vi "NK11003_Config.vi"(7 "频率":enum16{"50HZ", "60HZ"}(ring), 8 "error in":errorcluster caption="错误输入（无错误）", 9 "电流":dbl=10.0 min=1.0 max=13.0 format="%#_4f", 10 "电压":dbl=220.0 min=1.0 max=300.0 format="%#_4f", 11 "MyIndex":u8) -> (0 "error out":errorcluster, 3 "OK?":bool)   [LabVIEW 2015]
uses:
  <vilib>/Instr/_visa.llb/VISA Configure Serial Port (Instr).vi
panel:
  out "VISA":refnum<visa-resource-name> caption="VISA资源名称输出"
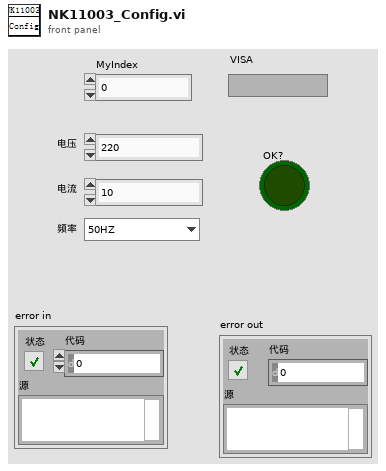
[diagram p1: front panel]
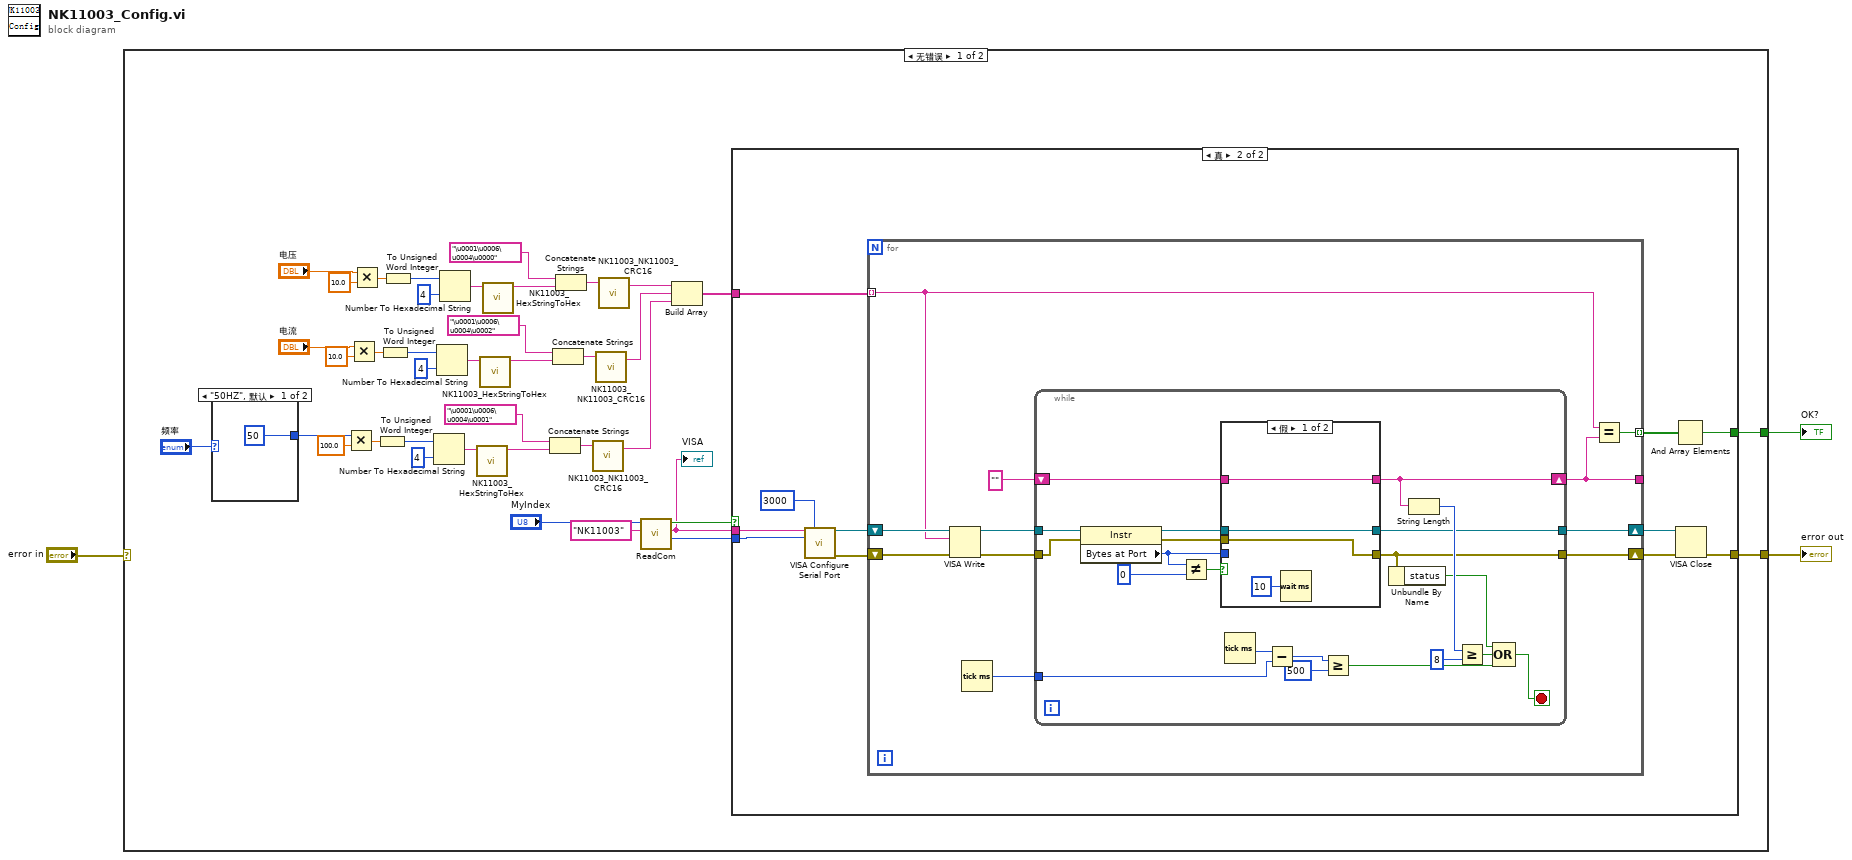
[diagram p0: block diagram]
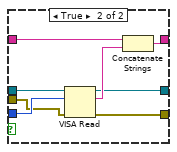
[diagram p3: hidden frame]
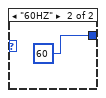
[diagram p4: hidden frame]
diagram:
  n1 = case shown="无错误" "error in" {
    selector: "error in" -> [_ w100]
    tunnel: [w8 _] -> w3
    tunnel: [w4 w100] -> w2
    frame No Error {
      n2 = case shown="\"50HZ\", 默认" "频率" {
        tunnel: [50 60] -> w14
        frame "50HZ", Default {
        }
        frame "60HZ" {
        }
      }
      n3 = Multiply(x=w14, y=100.0) -> (x*y=w21:dbl)
      n4 = Multiply(x="电流", y=10.0) -> (x*y=w27:dbl)
      n5 = Multiply(x="电压", y=10.0) -> (x*y=w38:dbl)
      n6 = To Unsigned Word Integer(number=w21) -> (unsigned 16bit integer=w20:u16)
      n7 = To Unsigned Word Integer(number=w27) -> (unsigned 16bit integer=w28:u16)
      n8 = To Unsigned Word Integer(number=w38) -> (unsigned 16bit integer=w37:u16)
      n9 = Number To Hexadecimal String(1:i16 4 ("宽度(-)"), 2:w20) -> (0:w18:string)
      n10 = Number To Hexadecimal String(1:i16 4 ("宽度(-)"), 2:w28) -> (0:w30:string)
      n11 = Number To Hexadecimal String(1:i16 4 ("宽度(-)"), 2:w37) -> (0:w35:string)
      n12 = call "NK11003_HexStringToHex.vi"("正常显示HEX字符串"=w18) -> ("HEX显示字符串"=w16:string)  [unwired: 10 in]
      n13 = call "NK11003_HexStringToHex.vi"("正常显示HEX字符串"=w30) -> ("HEX显示字符串"=w32:string)  [unwired: 10 in]
      n14 = call "NK11003_HexStringToHex.vi"("正常显示HEX字符串"=w35) -> ("HEX显示字符串"=w33:string)  [unwired: 10 in]
      n15 = Concatenate Strings("\u0001\u0006\u0004\u0001", w16) -> (w17:string)
      n16 = Concatenate Strings("\u0001\u0006\u0004\u0002", w32) -> (w31:string)
      n17 = Concatenate Strings("\u0001\u0006\u0004\u0000", w33) -> (w34:string)
      n18 = call "NK11003_NK11003_CRC16.vi"("input String"=w17) -> ("InPut +CRC"=w11:string)  [unwired: 1 out]
      n19 = call "NK11003_NK11003_CRC16.vi"("input String"=w31) -> ("InPut +CRC"=w12:string)  [unwired: 1 out]
      n20 = call "NK11003_NK11003_CRC16.vi"("input String"=w34) -> ("InPut +CRC"=w42:string)  [unwired: 1 out]
      n21 = call "ReadCom.vi"("仪器名称"="NK11003", "MyIndex"="MyIndex") -> ("Baudrate"=w6:i32, "COM"=w5:string, "OK?"=w7:bool)  [unwired: 7 in]
      "VISA" <- w5
      n22 = Build Array(w42, w12, w11) -> (w13:string[])
      n23 = case shown="真" w7 {
        tunnel: w13 -> [_ w49]
        tunnel: w5 -> [_ w47]
        tunnel: [_ w45] -> w8
        tunnel: w6 -> [_ w44]
        tunnel: [_ w43] -> w4
        frame False {
        }
        frame True {
          n24 = call-poly "VISA Configure Serial Port"("VISA resource name"=w47, "timeout (10sec)"=u32 3000, "baud rate (9600)"=w44) -> ("VISA resource name out"=w53:refnum<visa-resource-name>, "error out"=w52:errorcluster)  [unwired: 11 in]
          n25 = for {
            tunnel: [w56] -> _
            tunnel: w49 -> [w55] mode=indexing
            shift-right: [w58] -> w51
            shift-left: w53 -> [w64]
            shift-right: [w57] -> w50
            shift-left: w52 -> [w63]
            tunnel: [w54] -> w48 mode=indexing
            n26 = VISA Write(VISA resource name=w64, write buffer=w55, error in (no error)=w63) -> (VISA resource name out=w61:refnum<visa-resource-name>, error out=w62:errorcluster)  [unwired: 1 out]
            n27 = Tick Count (ms)() -> (millisecond timer value=w59:u32)
            n28 = while {
              tunnel: w62 -> [w65]
              tunnel: w61 -> [w85]
              shift-right: [w78] -> w56
              shift-left: "" -> [w79]
              tunnel: w59 -> [w71]
              tunnel: [w67] -> w58
              tunnel: [w66] -> w57
              stop <- w74 stop-if-true
              n29 = property class="Instr"(reference=w85, error in=w65) -> (reference out=w82:refnum<visa-resource-name>, error out=w80:errorcluster, "Bytes at Port"=w81:u32)
              n30 = Not Equal?(x=w81, y=u32 0) -> (x != y?=w83:bool)
              n31 = case shown="假" w83 {
                tunnel: w82 -> [w86 w97]
                tunnel: w81 -> [_ w96]
                tunnel: w80 -> [w87 w95]
                tunnel: w79 -> [w88 w94]
                tunnel: [w88 w92] -> w78
                tunnel: [w87 w91] -> w66
                tunnel: [w86 w90] -> w67
                frame False {
                  n32 = Wait (ms)(milliseconds to wait=u32 10 ("等待时间（毫秒）")) -> ()  [unwired: 1 out]
                }
                frame True {
                  n33 = VISA Read(VISA resource name=w97, byte count=w96, error in (no error)=w95) -> (VISA resource name out=w90:refnum<visa-resource-name>, read buffer=w93:string, error out=w91:errorcluster)  [unwired: 1 out]
                  n34 = Concatenate Strings(w94, w93) -> (w92:string)
                }
              }
              n35 = Tick Count (ms)() -> (millisecond timer value=w72:u32)
              n36 = Subtract(x=w72, y=w71) -> (x-y=w70:u32)
              n37 = Greater Or Equal?(x=w70, y=u32 500) -> (x >= y?=w68:bool)
              n38 = Unbundle By Name(w66) -> ("status"=w73:bool)
              n39 = String Length(string=w78) -> (length=w77:i32)
              n40 = Greater Or Equal?(x=w77, y=8) -> (x >= y?=w76:bool)
              n41 = Compound Arithmetic op=OR ("复合运算")(w73, w76, w68) -> (w74:bool)
            }
            n42 = Equal?(x=w55, y=w56) -> (x = y?=w54:bool)
          }
          n43 = And Array Elements(Boolean array=w48) -> (logical AND=w45:bool)
          n44 = VISA Close(VISA resource name=w51, error in (no error)=w50) -> (error out=w43:errorcluster)
        }
      }
    }
    frame Error {
    }
  }
  "OK?" <- w3
  "error out" <- w2
